vi "PathPlanner_PathFinder_WorkerThread.vi"() -> ()   [LabVIEW 2019, in "PathPlanner24.lvlib"]
uses:
  PathPlanner24.lvlib
  PathPlanner_GridPosition_New.vi
  PathPlanner_GridPosition_HashCode.vi
  PathPlanner_PathFinder_Constants.vi
  PathPlanner_PathFinder_Key.vi
  PathPlanner_PathFinder_OpenClear.vi
  PathPlanner_PathFinder_InconsClear.vi
  PathPlanner_PathFinder_ClosedClear.vi
  PathPlanner_PathFinder_ComputeOrImprovePath.vi
  PathPlanner_PathFinder_SetNewPathAvail.vi
  PathPlanner_PathFinder_ExtractPath.vi
  PathPlanner_GridPosition_Get.vi
  PathPlanner_PathFinder_Heuristic.vi
  PathPlanner_PathFinder_TopKey.vi
  PathPlanner_PathFinder_ComparePair.vi
  PathPlanner_PathFinder_UpdateState.vi
  PathPlanner_PathFinder_GetOpenNeighbors.vi
  PathPlanner_GridPosition_Equals.vi
  PathPlanner_GridPosition_FromHash.vi
  PathPlanner_PathFinder_IsWalkable.vi
  PathPlanner_PathFinder_GridPosToTranslation2d.vi
  <vilib>/Rock Robotics/WPI/ThirdParty/JAS_Junk/TrajLib/Translation2d_GetDistance.vi
  <vilib>/Rock Robotics/WPI/ThirdParty/JAS_Junk/TrajLib/Translation2d_Create_DistAng.vi
  <vilib>/Rock Robotics/WPI/ThirdParty/JAS_Junk/TrajLib/Translation2d_Minus.vi
  <vilib>/Rock Robotics/WPI/ThirdParty/JAS_Junk/TrajLib/Translation2d_GetAngle.vi
  <vilib>/Rock Robotics/WPI/ThirdParty/JAS_Junk/TrajLib/Translation2d_Plus.vi
  PathPlanner_PathFinder_Cost.vi
  <vilib>/Rock Robotics/WPI/ThirdParty/JAS_Junk/TrajLib/Translation2d_Create.vi
  <vilib>/Rock Robotics/WPI/ThirdParty/JAS_Junk/TrajLib/Util_CalcDist.vi
  <vilib>/Rock Robotics/WPI/ThirdParty/JAS_Junk/TrajLib/Rotation2d_GetAngleCosSin.vi
  <vilib>/Rock Robotics/WPI/ThirdParty/JAS_Junk/TrajLib/Translation2d_GetXY.vi
  <vilib>/Rock Robotics/WPI/ThirdParty/JAS_Junk/TrajLib/Rotation2d_CreateXY.vi
  PathPlanner_PathFinder_IsCollision.vi
  PathPlanner_PathFinder_Globals.vi
  PathPlanner_PathFinder_ApplyControlSmooth.vi
  PathPlanner_PathFinder_ApplyAnchorSmooth.vi
panel:
  in  "Main Name":string
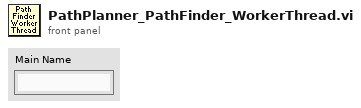
[diagram p1: front panel]
types:
  T1 = typedef "Semaphore RefNum" = refnum<k1>
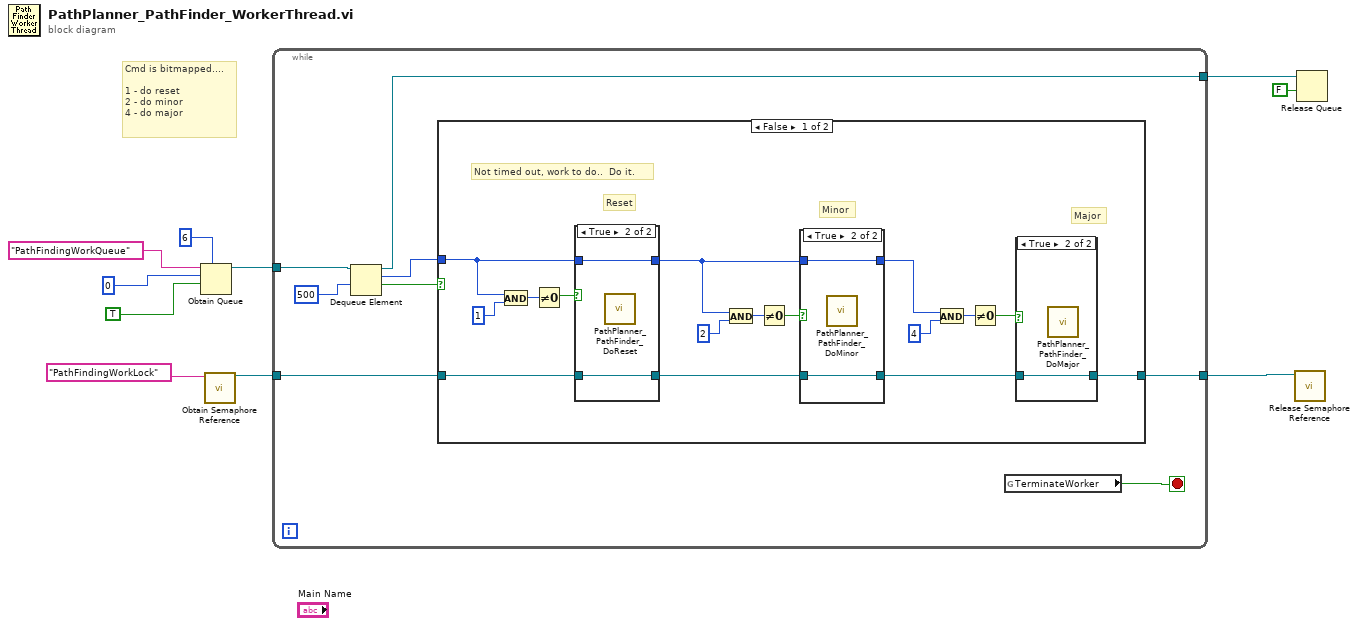
[diagram p0: block diagram]
diagram:
  # "Cmd is bitmapped....\n\n1 - do reset\n2 - do minor\n4 - do major"
  n1 = Obtain Queue(max queue size (-1, unlimited)=6, name (unnamed)="PathFindingWorkQueue", element data type=0, create if not found? (T)=TRUE) -> (queue out=w1:refnum<queue>)  [unwired: 1 in, 2 out]
  n2 = call <vilib>:"Obtain Semaphore Reference.vi"("name (unnamed)"="PathFindingWorkLock") -> ("semaphore"=w3:T1)  [unwired: 4 in, 2 out]
  n3 = while {
    tunnel: w1 -> [w17]
    tunnel: [w13] -> w6
    tunnel: w3 -> [w12]
    tunnel: [w11] -> w2
    stop <- w18 stop-if-true
    n4 = Dequeue Element(queue=w17, timeout in ms (-1)=500) -> (queue out=w13:refnum<queue>, element=w14:i32, timed out?=w15:bool)  [unwired: 1 in, 1 out]
    n5 = case shown="False" w15 {
      tunnel: w14 -> [w29 _]
      tunnel: w12 -> [w22 w45]
      tunnel: [w19 w45] -> w11
      frame False {
        # "Major"
        # "Minor"
        # "Reset"
        # "Not timed out, work to do..  Do it."
        n6 = And(x=w29, y=1) -> (x .and. y?=w32:i32)
        n7 = Not Equal To 0?(x=w32) -> (x != 0?=w33:bool)
        n8 = case shown="True" w33 {
          tunnel: w29 -> [w42 w44]
          tunnel: [w42 w44] -> w25
          tunnel: w22 -> [w41 w43]
          tunnel: [w41 w43] -> w21
          frame False {
          }
          frame True {
            n9 = call "PathPlanner_PathFinder_DoReset.vi"() -> ()  [unwired: 12 in]
          }
        }
        n10 = And(x=w25, y=2) -> (x .and. y?=w30:i32)
        n11 = Not Equal To 0?(x=w30) -> (x != 0?=w26:bool)
        n12 = case shown="True" w26 {
          tunnel: w25 -> [w38 w40]
          tunnel: [w38 w40] -> w23
          tunnel: w21 -> [w37 w39]
          tunnel: [w37 w39] -> w20
          frame False {
          }
          frame True {
            n13 = call "PathPlanner_PathFinder_DoMinor.vi"() -> ()  [unwired: 12 in]
          }
        }
        n14 = And(x=w23, y=4) -> (x .and. y?=w27:i32)
        n15 = Not Equal To 0?(x=w27) -> (x != 0?=w24:bool)
        n16 = case shown="True" w24 {
          tunnel: w20 -> [w35 w36]
          tunnel: [w35 w36] -> w19
          frame False {
          }
          frame True {
            n17 = call "PathPlanner_PathFinder_DoMajor.vi"() -> ()  [unwired: 12 in]
          }
        }
      }
      frame True {
        # "#TODO  Add I'm alive counter"
        # "Timed out, no work to do...."
      }
    }
    n18 = global read "PathPlanner_PathFinder_Globals.vi" "TerminateWorker"() -> (w18:bool)
  }
  n19 = call <vilib>:"Release Semaphore Reference.vi"("semaphore"=w2) -> ()  [unwired: 9 in, 2 out]
  n20 = Release Queue(queue=w6, force destroy? (F)=FALSE) -> ()  [unwired: 1 in, 3 out]
